vi "FTW-CodeGen-GenerateCode.vi"(0 "State In":T2, 5 "XRef":refnum<vi>, 7 "Terms":T1(array[cluster]), 9 "Diagram":refnum<vi>) -> (4 "State Out":T2, 6 "Reply":string[](array[string]), 8 "Generated Code?":bool)   [LabVIEW 2014, in "FTW-JSON-Deserialize.xnode"]
uses:
  FTW-JSON-Deserialize.xnode
  FTW-CodeGen-State.ctl
  codegen/FTW-CodeGen-XNodeReplyType.ctl
  FTW-CodeGen-Prototype.vi
panel:
  # "Inputs"
  # "Outputs"
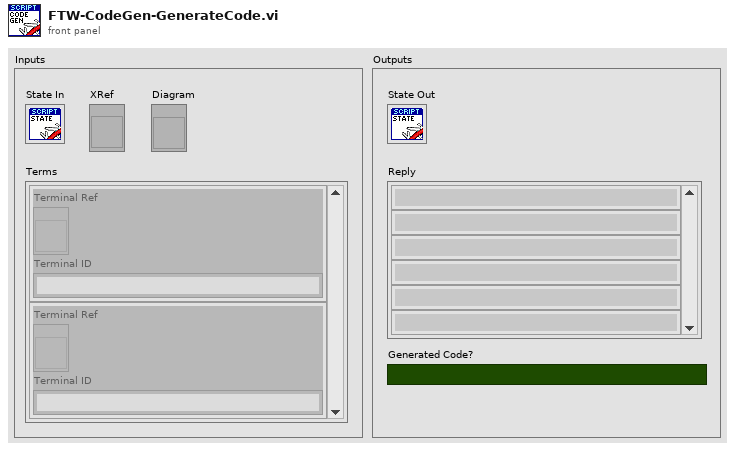
[diagram p1: front panel]
types:
  T1 = cluster{"Terminal Ref":refnum<vi>, "Terminal ID":string}[]
  T2 = typedef "FTW-JSON-Deserialize.xnode/FTW-CodeGen-State.ctl" = cluster{"Dummy":string}
  T3 = typedef "FTW-CodeGen-XNodeReplyType.ctl" = enum16{"UpdateState", "AdaptToInputs", "AdaptAndAugment", "CosmeticUpdate", "NoReply"}
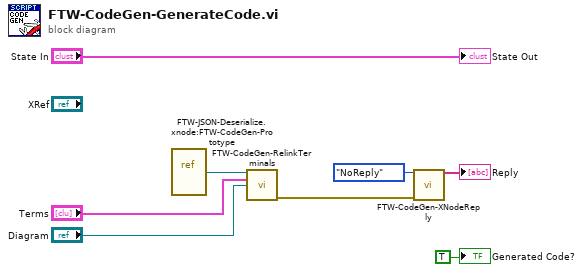
[diagram p0: block diagram]
diagram:
  n1 = vi-ref "FTW-JSON-Deserialize.xnode:FTW-CodeGen-Prototype.vi"() -> (w6:refnum<vi>)
  n2 = call "FTW-CodeGen-RelinkTerminals.vi"("PrototypeVI"=w6, "Terms"="Terms", "Diagram"="Diagram") -> ("error out"=w3:errorcluster)  [unwired: 12 in]
  n3 = call "FTW-CodeGen-XNodeReply.vi"("XNode Reply Type"=FTW-CodeGen-XNodeReplyType."NoReply", "error in"=w3) -> ("Reply"=→"Reply":string[])  [unwired: 13 in]
  "State Out" <- "State In"
  "Generated Code?" <- TRUE ("Generated Code?")
